vi "SetAngleUnits.vi"(8 "error in":errorcluster, 11 "UnitName":string) -> (0 "error out":errorcluster)   [LabVIEW 2013]
uses:
  CRCL Globals.vi
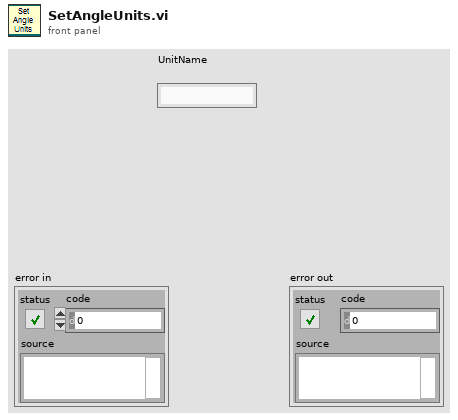
[diagram p1: front panel]
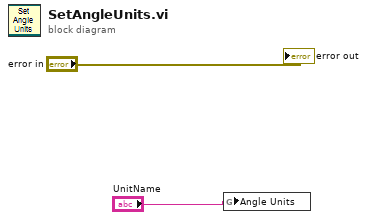
[diagram p0: block diagram]
diagram:
  n1 = global write "CRCL Globals.vi" "Angle Units"("UnitName") -> ()
  "error out" <- "error in"
